vi "Unpack Message.vi"(8 "error in (no error)":errorcluster, 9 "Packed Message":string, 10 "Message Name":string, 11 "Message Double in":refnum<class "Message Double and Boolean Array.lvclass">) -> (0 "error out":errorcluster, 2 "Valid":bool, 3 "Message Double out":refnum<class "Message Double and Boolean Array.lvclass">)   [LabVIEW 2016, in "WebSocket Networking.lvlib" / "Message Double and Boolean Array.lvclass"]
uses:
  <userlib>/Common Components/WebSocket Networking/Message Double and Boolean Array/Message Double and Boolean Array.lvclass
  C:/Program Files (x86)/National Instruments/LabVIEW 2016/user.lib/Composed Systems/Stream/Mediator/Classes/Message Interface/Message Interface.lvclass
  <userlib>/Common Components/WebSocket Networking/Message Double and Boolean Array/Value.ctl
  <userlib>/Common Components/WebSocket Networking/Message Double and Boolean Array/Message Double and Boolean Array.lvclass/Message Double and Boolean Array.ctl
  <userlib>/Composed Systems/Stream/Mediator/Classes/Message Interface/Message Interface.lvclass
  <vilib>/addons/_JKI.lib/Serialization/JSON/JKI JSON Serialization.lvlib
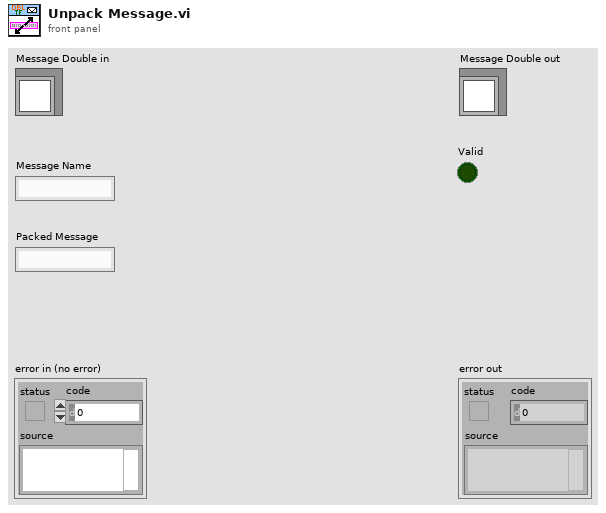
[diagram p1: front panel]
types:
  T1 = typedef "WebSocket Networking.lvlib/Message Double and Boolean Array.lvclass/Value.ctl" = cluster{"Master ID":string, "Doubles":dbl[], "Booleans":bool[]}
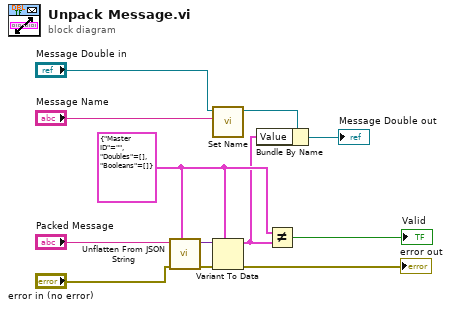
[diagram p0: block diagram]
diagram:
  w3 = T1 {"Master ID"="", "Doubles"=[], "Booleans"=[]} ("Value")
  n1 = call <vilib>:"Unflatten From JSON String.vi"("Type and Defaults"=w3, "error in (no error)"="error in (no error)", "JSON String"="Packed Message") -> ("error out"=w6:errorcluster, "Variant"=w8:variant)  [unwired: 7 in]
  n2 = call <userlib>:"Set Name.vi"("Name"="Message Name", "Message Interface in"="Message Double in") -> ("Message Interface out"=w10:refnum<class "Message Double and Boolean Array.lvclass">)  [unwired: 8 in, 1 out]
  n3 = Variant To Data(error in=w6, type=w3, Variant=w8) -> (data=w2:T1, error out=→"error out":errorcluster)
  n4 = Bundle By Name(cluster=w10, "Value"=w2) -> (→"Message Double out":refnum<class "Message Double and Boolean Array.lvclass">)
  n5 = Not Equal?(x=w3, y=w2) -> (x != y?=→"Valid":bool)
